vi "Read Absolute Delay.vi"(11 "Abstract Delay Line in":refnum<class "Abstract Delay Line.lvclass">) -> (2 "Absolute Delay (ps)":i32, 3 "Abstract Delay Line out":refnum<class "Abstract Delay Line.lvclass">)   [LabVIEW 2016, in "Delay Line.lvlib" / "Abstract Delay Line.lvclass"]
uses:
  Abstract Delay Line.lvclass
  Abstract Delay Line.lvclass/Abstract Delay Line.ctl
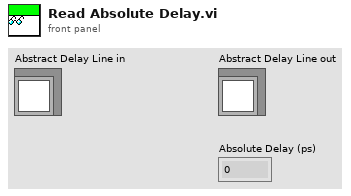
[diagram p1: front panel]
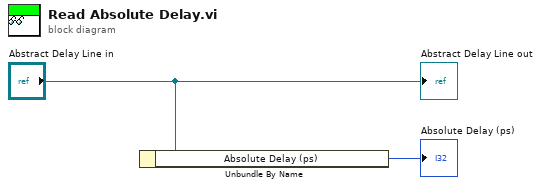
[diagram p0: block diagram]
diagram:
  n1 = Unbundle By Name("Abstract Delay Line in") -> ("Absolute Delay (ps)"=→"Absolute Delay (ps)":i32)
  "Abstract Delay Line out" <- "Abstract Delay Line in"
